vi "DAQmx Task Name.vi"(1 "DAQmx Task Name":refnum<k21>) -> (0 "DAQmx Task Name Out":refnum<k21>)   [LabVIEW 2012]
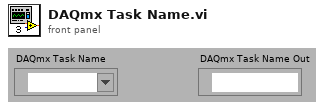
[diagram p1: front panel]
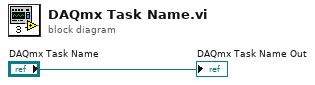
[diagram p0: block diagram]
diagram:
  "DAQmx Task Name Out" <- "DAQmx Task Name"
